vi "Test Different ImageResIDs.vi"(8 "error in (no error)":errorcluster) -> (0 "error out":errorcluster)   [LabVIEW 2026, in "VILab.lvlib"]
uses:
  VILab.lvlib
  SubVIs/Find Resource by Type (String).vi
  CTLs/Resource.ctl
  <vilib>/Utility/traverseref.llb/VI Scripting - Traverse.lvlib
  <vilib>/Utility/traverseref.llb/TRef TravTarget.ctl
panel:
  out "Last Error":errorcluster
  out "Working IDs":i32[](array[numeric])=[0, 1, 2, 3, 4, 5, 6, 7, 8, 9, 10, 11, 12, 13, 14, 15, 16, 17, 18, 19, 20, 21, 22, 23, 24, 25, 26, 27, 28, 29, 30, 31, 32, 33, 34, 35, 36, 37, 38, 39, 40, 41, 42, 43, 44, 45, 46, 47, 48, 49, 50, 51, 52, 53, 54, 55, 56, 57, 58, 59, 60, 61, 62, 63, 64, 65, 66, 67, 68, 69, 70, 71, 72, 73, 74, 75, 76, 77, 78, 79, 80, 81, 82, 83, 84, 85, 86, 87, 88, 89, 90, 91, 92, 93, 94, 95, 96, 97, 98, 99, 100, 101, 102, 103, 104, 105, 106, 107, 108, 109, 110, 111, 112, 113, 114, 115, 116, 117, 118, 119, 120, 121, 122, 123, 124, 125, 126, 127, 128, 129, 130, 131, 132, 133, 134, 135, 136, 137, 138, 139, 140, 141, 142, 143, 144, 145, 146, 147, 148, 149, 150, 151, 152, 153, 154, 155, 156, 157, 158, 159, 160, 161, 162, 163, 164, 165, 166, 167, 168, 169, 170, 171, 172, 173, 174, 175, 176, 177, 178, 179, 180, 181, 182, 183, 184, 185, 186, 187, 188, 189, 190, 191, 192, 193, 194, 195, 196, 197, 198, 199, 200, 201, 202, 203, 204, 205, 206, 207, 208, 209, 210, 211, 212, 213, 214, 215, 216, 217, 218, 219, 220, 221, 222, 223, 224, 225, 226, 227, 228, 229, 230, 231, 238, 239, 240, 241, 242, 243, 244, 245, 246, 247, 248, 249, 250, 251, 252, 253, 254, 255, 256, 257, 258, 259, 260, 261, 262, 263, 264, 265, 266, 267, 268, 269, 270, 271, 272, 273, 274, 275, 276, 277, 278, 279, 280, 281, 282, 283, 284, 285, 286, 287, 288, 289, 290, 291, 292, 293, 294, 295, 296, 297, 298, 299, 300, 301, 302, 303, 304, 305, 306, 307, 308, 309, 310, 311, 312, 313, 314, 315, 316, 317, 318, 319, 320, 321, 322, 323, 324, 325, 326, 327, 328, 329, 330, 331, 332, 333, 334, 335, 336, 337, 338, 339, 340, 341, 342, 343, 344, 345, 346, 347, 348, 349, 350, 351, 352, 353, 354, 355, 356, 357, 358, 359, 360, 361, 362, 363, 364, 365, 366, 373, 374, 375, 376, 377, 378, 379, 380, 381, 382, 383, 384, 385, 386, 387, 388, 389, 390, 391, 393, 394, 395, 396, 397, 398, 399, 400, 401, 402, 403, 404, 405, 406, 407, 408, 409, 410, 411, 412, 413, 414, 415, 416, 417, 418, 419, 420, 421, 422, 423, 424, 425, 426, 427, 428, 429, 430, 431, 432, 433, 434, 435, 436, 437, 438, 439, 440, 441, 442, 443, 444, 445, 446, 447, 448, 449, 450, 451, 452, 453, 454, 455, 456, 457, 458, 459, 460, 461, 462, 463, 464, 465, 466, 467, 468, 469, 470, 471, 472, 473, 474, 475, 476, 477, 478, 479, 480, 481, 482, 483, 484, 485, 486, 487, 488, 489, 490, 491, 492, 493, 494, 495, 496, 497, 498, 499, 500, 505, 506, 507, 508, 509, 510, 511, 512, 513, 514, 515, 516, 517, 518, 519, 520, 521, 522, 523, 524, 525, 526, 527, 528, 529, 530, 531, 533, 534, 535, 536, 537, 538, 539, 540, 541, 543, 544, 545, 546, 547, 548, 549, 550, 551, 552, 553, 554, 555, 556, 557, 558, 559, 560, 561, 562, 563, 564, 565, 566, 567, 568, 569, 570, 571, 572, 573, 574, 575, 576, 577, 578, 579, 580, 581, 582, 583, 584, 585, 586, 587, 588, 589, 590, 591, 592, 593, 594, 595, 596, 597, 598, 599, 600, 601, 602, 603, 604, 605, 606, 607, 608, 609, 610, 611, 612, 613, 614, 615, 616, 617, 618, 619, 620, 621, 622, 623, 624, 625, 626, 627, 628, 629, 630, 631, 632, 633, 634, 635, 636, 637, 638, 639, 640, 641, 644, 645, 648, 649, 650, 651, 652, 653, 654, 655, 656, 657, 658, 659, 660, 661, 662, 663, 664, 665, 666, 667, 668, 669, 670, 671, 672, 673, 674, 675, 676, 677, 678, 679, 680, 681, 682, 683, 684, 685, 686, 687, 688, 689, 690, 691, 692, 693, 694, 695, 696, 697, 698, 699, 700, 701, 702, 703, 704, 705, 706, 707, 708, 709, 710, 711, 712, 713, 714, 715, 716, 717, 718, 719, 720, 721, 722, 723, 724, 725, 726, 727, 728, 729, 730, 731, 732, 733, 734, 735, 736, 737, 738, 739, 740, 741, 742, 743, 744, 745, 746, 747, 748, 749, 750, 751, 752, 753, 754, 755, 756, 757, 758, 759, 760, 761, 762, 763, 764, 766, 767, 768, 769, 771, 772, 773, 774, 775, 776, 777, 778, 779, 780, 781, 782, 783, 786, 787, 788, 789, 790, 791, 792, 793, 794, 795, 796, 797, 798, 799, 800, 801, 802, 803, 804, 805, 806, 807, 808, 809, 810, 811, 812, 813, 814, 815, 816, 817, 818, 819, 820, 821, 822, 823, 824, 825, 826, 827, 828, 829, 830, 831, 832, 833, 834, 835, 836, 837, 838, 839, 1000, 1001, 1002, 1003, 1004, 1005, 1006, 1007, 1008, 1009, 1010, 1011, 1012, 1013, 1014, 1015, 1016, 1017, 1018, 1019, 1020, 1021, 1022, 1023, 1024, 1025, 1026, 1027, 1028, 1029, 1030, 2000, 2001, 2002, 2003, 2004, 2005, 2006, 2007, 2008, 2009, 2010, 2011, 2012, 2013, 2014, 2015, 2016, 2017, 2018, 2019, 2020, 2021, 2022, 2023, 2024, 2025, 2026, 2027, 2028, 2029, 2030, 2031, 2032, 2033, 2034, 2035, 2036, 2037, 2038, 2039, 2040, 2041, 2042, 2043, 2044, 2045, 2046, 2047, 2048, 2049, 2050, 2051, 2052, 2053, 2054, 2055, 2056, 2057, 2058, 2059, 2060, 2061, 2062, 2063, 2064, 2065, 2066, 2067, 2068, 2069, 2070, 2071, 2072, 2073, 2074, 2075, 2076, 2077, 2078, 2079, 2080, 2081, 2082, 2083, 2084, 2085, 2086, 2087, 2088, 2089, 2090, 2091, 2092, 2093, 2094, 2095, 2096, 2097, 2098, 2099, 2100, 2101, 2102, 2103, 2104, 2105, 2106, 2107, 2108, 2109, 3000, 3001, 3002, 3003, 3004, 3005, 3006, 3007, 3008, 3009, 3010, 3011, 3012, 3013, 3014, 3015, 3016, 3017, 3018, 3019, 3020, 3021, 3022, 3023, 3024, 3025, 3026, 3027, 3028, 3029, 3030, 3031, 3032, 3033, 3034, 3035, 3036, 3037, 3038, 3039, 3040, 3041, 3042, 3043, 3044, 3045, 3046, 3047, 3048, 3049, 3050, 3051, 3052, 3053, 3054, 3055, 3056, 3057, 3058, 3059, 3060, 3061, 3062, 3063, 3064, 3065, 3066, 3067, 3068, 3069, 3070, 3071, 3072, 3073, 3074, 3075, 3076, 3077, 3078, 3079, 3080, 3081, 3082, 3083, 3084, 3085, 3086, 3087, 3088, 3089, 3090, 3091]
  out "i":i32
  in  "stop":bool
  # "tried up to -5000"
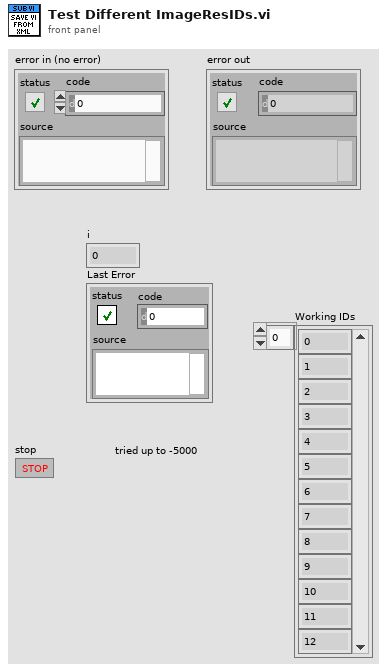
[diagram p1: front panel]
types:
  T1 = typedef "TRef TravTarget.ctl" = enum16{"FP", "BD", "Other"}
  T2 = typedef "VILab.lvlib/Resource.ctl" = cluster{"type":u32, "id":i32, "name":string, "binary data":string}
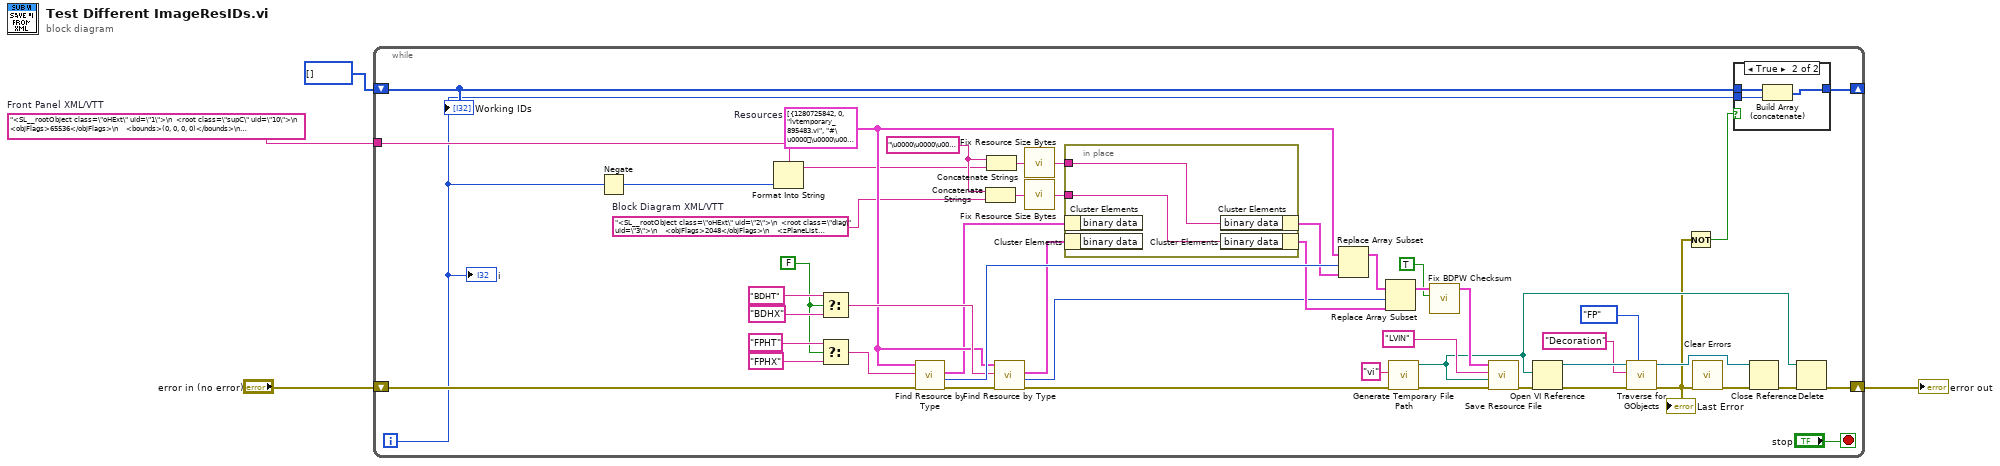
[diagram p0: block diagram]
diagram:
  w2 = "<SL__rootObject class=\"oHExt\" uid=\"1\">\n  <root class=\"supC\" uid=\"10\">\n    <objFlags>65536</objFlags>\n    <bounds>(0, 0, 0, 0)</bounds>\n    <MouseWheelSupport>0</MouseWheelSupport>\n    <ddoList elements=\"0\">\n      </ddoList>\n    <paneHierarchy class=\"pane\" uid=\"12\">\n      <objFlags>2492464</objFlags>\n      <howGrow>240</howGrow>\n      <bounds>(46, 0, 668, 1090)</bounds>\n      <partsList elements=\"6\">\n        <SL__arrayElement class=\"label\" uid=\"15\">\n          <objFlags>1511754</objFlags>\n          <partID>16</partID>\n          <masterPart>28</masterPart>\n          <howGrow>5</howGrow>\n          <bounds>(0, 0, 17, 29)</bounds>\n          <image class=\"Image\">\n            <ImageResID>-9</ImageResID>\n            </image>\n          <fgColor>01000000</fgColor>\n          <bgColor>01000000</bgColor>\n          <textRec class=\"textHair\">\n            <mode>1028</mode>\n            <text>\"Pane\"</text>\n            <bgColor>01000000</bgColor>\n            </textRec>\n          </SL__arrayElement>\n        <SL__arrayElement class=\"cosm\" uid=\"16\">\n          <objFlags>3442</objFlags>\n          <partID>39</partID>\n          <masterPart>28</masterPart>\n          <howGrow>194</howGrow>\n          <bounds>(0, 1073, 605, 1090)</bounds>\n          <image class=\"Image\">\n            <ImageResID>0</ImageResID>\n            </image>\n          <bgColor>00B3B3B3</bgColor>\n          </SL__arrayElement>\n        <SL__arrayElement class=\"cosm\" uid=\"17\">\n          <objFlags>3442</objFlags>\n          <partID>38</partID>\n          <masterPart>28</masterPart>\n          <howGrow>56</howGrow>\n          <bounds>(605, 0, 622, 1073)</bounds>\n          <image class=\"Image\">\n            <ImageResID>0</ImageResID>\n            </image>\n          <bgColor>00B3B3B3</bgColor>\n          </SL__arrayElement>\n        <SL__arrayElement class=\"cosm\" uid=\"18\">\n          <objFlags>7539</objFlags>\n          <partID>44</partID>\n          <masterPart>28</masterPart>\n          <howGrow>10</howGrow>\n          <bounds>(605, 1073, 622, 1090)</bounds>\n          <image class=\"Image\">\n            <ImageResID>-365</ImageResID>\n            </image>\n          <fgColor>00B3B3B3</fgColor>\n          <bgColor>00B3B3B3</bgColor>\n          </SL__arrayElement>\n        <SL__arrayElement class=\"cosm\" uid=\"19\">\n          <objFlags>4211</objFlags>\n          <partID>28</partID>\n          <howGrow>120</howGrow>\n          <bounds>(0, 0, 605, 1073)</bounds>\n          <image class=\"Image\">\n            <ImageResID>-704</ImageResID>\n            </image>\n          <fgColor>00E2E2E2</fgColor>\n          <bgColor>00E2E2E2</bgColor>\n          </SL__arrayElement>\n        <SL__arrayElement class=\"annex\" uid=\"20\">\n          <partID>66</partID>\n          </SL__arrayElement>\n        </partsList>\n      <paneFlags>331089</paneFlags>\n      <minPaneSize>(1,1)</minPaneSize>\n      <docBounds>(-127, -244, 605, 1073)</docBounds>\n      <zPlaneList elements=\"1\">\n        <SL__arrayElement class=\"cosm\" uid=\"52\">\n          <objFlags>3</objFlags>\n          <bounds>(-22, 24, 10, 56)</bounds>\n          <image class=\"Image\">\n            <ImageResID>%d</ImageResID>\n            </image>\n          <fgColor>00A8ABAE</fgColor>\n          <bgColor>00FFFFFF</bgColor>\n          </SL__arrayElement>\n        </zPlaneList>\n      <image class=\"Image\">\n        <ImageResID>0</ImageResID>\n        </image>\n      </paneHierarchy>\n    <savedSize>(0, 0, 0, 0)</savedSize>\n    <conPane class=\"conPane\" uid=\"21\">\n      <conId>4815</conId>\n      <cons elements=\"12\">\n        </cons>\n      </conPane>\n    <keyMappingList class=\"keyMapList\" uid=\"22\">\n      </keyMappingList>\n    </root>\n  <pBounds>(46, 0, 668, 1090)</pBounds>\n  <dBounds>(0, 0, 0, 0)</dBounds>\n  <origin>(723,351)</origin>\n  <instrStyle>31</instrStyle>\n  <blinkList elements=\"0\">\n    </blinkList>\n  </SL__rootObject>\n"  # Front Panel XML/VTT
  n1 = while {
    shift-right: [w13] -> w3
    shift-left: "error in (no error)" -> [w30]
    tunnel: w2 -> [w24]
    shift-right: [w20] -> _
    shift-left: i32[] [] -> [w22]
    i -> [w21]
    stop <- "stop" stop-if-true
    w28 = FALSE ("Use VTT?")
    w26 = "<SL__rootObject class=\"oHExt\" uid=\"2\">\n  <root class=\"diag\" uid=\"3\">\n    <objFlags>2048</objFlags>\n    <zPlaneList elements=\"0\">\n      </zPlaneList>\n    <nodeList elements=\"1\">\n      <SL__arrayElement class=\"sRN\" uid=\"7\">\n        <termList elements=\"0\">\n          </termList>\n        <bounds>(0, 0, 0, 0)</bounds>\n        <shortCount>1</shortCount>\n        <clumpNum>131075</clumpNum>\n        </SL__arrayElement>\n      </nodeList>\n    <signalList elements=\"0\">\n      </signalList>\n    <bgColor>00FFFFFF</bgColor>\n    <firstNodeIdx>1</firstNodeIdx>\n    </root>\n  <pBounds>(46, 0, 651, 1073)</pBounds>\n  <dBounds>(46, 0, 651, 1073)</dBounds>\n  <origin>(1124,436)</origin>\n  <instrStyle>31</instrStyle>\n  </SL__rootObject>\n"  # Block Diagram XML/VTT
    w27 = T2[] [{"type"=1280725842, "id"=0, "name"="lvtemporary_895483.vi", "binary data"="#\u0000\u0000\u0000\u0000\u0000\u0000 \u0000\u0006\u0000\u0000\u0000\u0000\u0004\u0000\u0003\u0000<\u0000\u0000\u0000\u001f@\u0002\u0000\u0000\u0000\u0000\u0001\u0000\u0001\u0000\u0002ÿÿÿÿ\u0000\u0000\u0000\u0000\u0000\u0000\u0000\u0000\u0000\u0000\u0000\u0000\u0000\u0000\u0000\u0000\u0000\u0000\u0000\u0000\u0000\u0000\u0000\u0000\u0000\u0000\u0000\u0000\u0000\u0000\u0000\f\u0000\u0000\u0000\u0010\u0000\u0000\u0000\u0000\u0000\u0000\u0000\u0000\u0000\u0000\u0000\u0000\u0000\u0000\u0000\u0000\u0000\u0000\u0000\u0000Ô\u001dÙ\u0000²\u0004é\tìøB~\u0000\u0000\u0000\u0000\u0000\u0000\u0000\u0000\u0000\u0000\u0000\u0000\u0000\u0000\u0000\u0000\u0000\u0000\u0000\u0000\u0000\u0000\u0000\u0000\u0001\u0000\u0000\u0000ÿÿÿÿÔ\u001dÙ\u0000²\u0004é\tìøB~"}, {"type"=1381258055, "id"=0, "name"="", "binary data"="\u0000\u0000\u0000\u0000\u0000\u0000\u0000\u0000\u0000\u0000\u0000\u0000\u0000\u0000\u0000\u0000"}, {"type"=1986359923, "id"=4, "name"="", "binary data"="#6€\u0006\u0000\u0000\u000623.3.6\u0000"}, {"type"=1129270864, "id"=0, "name"="", "binary data"="\u0000\u0001"}, {"type"=1279882857, "id"=0, "name"="", "binary data"="\u0000\u0001LVIN\u0000\u0000\u0000\u0000\u0000\u0003"}, {"type"=1111773271, "id"=0, "name"="", "binary data"="Ô\u001dÙ\u0000²\u0004é\tìøB~K@I.b\u0001-\u001amå­U\u0006òv\u001f\n¦©fí²\u0002\u0013@î¼ "}, {"type"=1229147982, "id"=0, "name"="", "binary data"="ÿÿÿÿ\u0000\u0000\u0001\u0000\u0000\u0001ÿü\u0001\u0000T\u0001ÿT\u0001ûT\u0001u\u0004\u0001u$\u0001®T\u0001®T\u0001ß$\u0001ÿ\u0004\u0001\u0000\u001c\u0001\u0000\u0016\u0001\u0010ñ;\u0012a$\u0017\u001dÿòaIñ2\u0016\u0001\u0018\u0001x\u0000\u0001\u0000\u0000\u0001\u0000\u0000\u0001\u0000\u0000\u0001\u0000\u0000\u0001\u0000\u0000\u0001\u0000\u0000\u0001\u0000\u0000\u0001\u0000\u0000\u0001ÿÿÿÿ"}, {"type"=1768123448, "id"=0, "name"="", "binary data"="ÿÿÿÿÿÿÿÿÿÿÿÿÿÿÿÿÿÿÿÿÿÿÿÿÿÿÿÿÿÿÿÿÿ\u0000\u0000\u0000\u0000\u0000\u0000\u0000\u0000\u0000\u0000\u0000\u0000\u0000\u0000\u0000\u0000\u0000\u0000\u0000\u0000\u0000\u0000\u0000\u0000\u0000\u0000\u0000\u0000\u0000\u0000ÿÿ\u0000\u0000\u0000\u0000\u0000\u0000\u0000\u0000\u0000\u0000\u0000\u0000\u0000\u0000\u0000\u0000\u0000\u0000\u0000\u0000\u0000\u0000\u0000\u0000\u0000\u0000\u0000\u0000\u0000\u0000ÿÿ\u0000\u0000ÿÿÿÿÿÿÿÿÿÿÿÿÿÿÿÿÿÿÿ\u0000\u0000\u0000\u0000\u0000\u0000\u0000\u0000\u0000ÿÿ\u0000\u0000ÿùùùùùùùùùùùù÷ù,ù,à\u0000\u0000\u0000\u0000\u0000\u0000\u0000\u0000\u0000ÿÿ\u0000\u0000ÿùÿÿÿÿÿÿÿÿÿÿÿ÷ù,ù,ÿ\u0000\u0000\u0000\u0000\u0000\u0000\u0000\u0000\u0000ÿÿ\u0000\u0000ÿùÿèäèÿÿÿèäèÿ÷ü+ü,ÿ\u0000\u0000\u0000\u0000\u0000\u0000\u0000\u0000\u0000ÿÿ\u0000\u0000ÿùÿäÿäÿÿÿäÿäÿ÷,,,,à\u0000\u0000\u0000\u0000\u0000\u0000\u0000\u0000\u0000ÿÿ\u0000\u0000ÿùèäÿäèÿèäÿäè÷+ü+,ÿ\u0000\u0000\u0000\u0000\u0000\u0000\u0000\u0000\u0000ÿÿ\u0000\u0000ÿùäèÿèäÿäèÿèä÷ü\bü,ÿ\u0000\u0000\u0000\u0000\u0000\u0000\u0000\u0000\u0000ÿÿ\u0000\u0000ÿùäÿÿÿäÿäÿÿÿä÷ü\bü,ÿ\u0000\u0000\u0000\u0000\u0000\u0000\u0000\u0000\u0000ÿÿ\u0000\u0000ÿùÿÿÿÿèäèÿÿÿÿ÷+ü+,ÿ\u0000\u0000\u0000\u0000\u0000\u0000\u0000\u0000\u0000ÿÿ\u0000\u0000ÿùÿÿÿÿÿÿÿÿÿÿÿ÷,,,,ÿ\u0000\u0000\u0000\u0000\u0000\u0000\u0000\u0000\u0000ÿÿ\u0000\u0000ÿ÷÷÷÷÷÷÷÷÷÷÷÷÷,,ƒƒÿ\u0000\u0000\u0000\u0000\u0000\u0000\u0000\u0000\u0000ÿÿ\u0000\u0000ÿ,,,,,,,,,,,,,,,ƒ\u0005ƒƒ\u0000\u0000\u0000\u0000\u0000\u0000\u0000\u0000ÿÿ\u0000\u0000ÿ,ü,,,,,ü,,,,###ƒ\u0005\u0005\u0005ƒƒ\u0000\u0000\u0000\u0000\u0000\u0000ÿÿ\u0000\u0000ÿüðü,,,ü#ü,##,,,ƒ\u0005\u0005ÿ\u0005\u0005ƒƒ\u0000\u0000\u0000\u0000ÿÿ\u0000\u0000ÿ,ï,,,,#,,#,,,,,ƒ\u0005ÿÿÿ\u0005\u0005\u0005ƒ##\u0000ÿÿ\u0000\u0000ÿÿðÿÿÿ#ÿÿ#ÿÿÿÿÿÿƒ\u0005\u0005ÿ\u0005..."}, {"type"=1414091852, "id"=0, "name"="", "binary data"="\tSource VI"}, {"type"=1129333554, "id"=0, "name"="", "binary data"="\u0000\u0001"}, {"type"=1279878768, "id"=0, "name"="", "binary data"="\u0000\u0001FPHP\u0000\u0000\u0000\u0000\u0000\u0003"}, {"type"=1179665784, "id"=0, "name"="", "binary data"="\u0000\u0000\u0000\u0000"}, {"type"=1179666520, "id"=0, "name"="", "binary data"="\u0000\u0000\u000eØ<SL__rootObject class=\"oHExt\" uid=\"1\">\n  <root class=\"supC\" uid=\"10\">\n    <objFlags>65536</objFlags>\n    <bounds>(0, 0, 0, 0)</bounds>\n    <MouseWheelSupport>0</MouseWheelSupport>\n    <ddoList elements=\"0\">\n      </ddoList>\n    <paneHierarchy class=\"pane\" uid=\"12\">\n      <objFlags>2492464</objFlags>\n      <howGrow>240</howGrow>\n      <bounds>(46, 0, 668, 1090)</bounds>\n      <partsList elements=\"6\">\n        <SL__arrayElement class=\"label\" uid=\"15\">\n          <objFlags>1511754</objFlags>\n          <partID>16</partID>\n          <masterPart>28</masterPart>\n          <howGrow>5</howGrow>\n          <bounds>(0, 0, 17, 29)</bounds>\n          <image class=\"Image\">\n            <ImageResID>-9</ImageResID>\n            </image>\n          <fgColor>01000000</fgColor>\n          <bgColor>01000000</bgColor>\n          <textRec class=\"textHair\">\n            <mode>1028</mode>\n            <text>\"Pane\"</text>\n            <bgColor>01000000</bgColor>\n            </textRec>\n          </SL__arrayElement>\n        <SL__arrayElement class=\"cosm\" uid=\"16\">\n          <objFlags>3442</objFlags>\n          <partID>39</partID>\n          <masterPart>28</masterPart>\n          <howGrow>194</howGrow>\n          <bounds>(0, 1073, 605, 1090)</bounds>\n          <image class=\"Image\">\n            <ImageResID>0</ImageResID>\n            </image>\n          <bgColor>00B3B3B3</bgColor>\n          </SL__arrayElement>\n        <SL__arrayElement class=\"cosm\" uid=\"17\">\n          <objFlags>3442</objFlags>\n          <partID>38</partID>\n          <masterPart>28</masterPart>\n          <howGrow>56</howGrow>\n          <bounds>(605, 0, 622, 1073)</bounds>\n          <image class=\"Image\">\n            <ImageResID>0</ImageResID>\n            </image>\n          <bgColor>00B3B3B3</bgColor>\n          </SL__arrayElement>\n        <SL__arrayElement class=\"cosm\" uid=\"18\">\n          <objFlags>7539</objFlags>\n          <partID>44</partID>\n          <masterPart>28</masterPart>\n          <howGrow>10</howGrow>\n          <bounds>(605, 1073, 622, 1090)</bounds>\n          <image class=\"Image\">\n            <ImageResID>-365</ImageResID>\n            </image>\n          <fgColor>00B3B3B3</fgColor>\n          <bgColor>00B3B3B3</bgColor>\n          </SL__arrayElement>\n        <SL__arrayElement class=\"cosm\" uid=\"19\">\n          <objFlags>4211</objFlags>\n          <partID>28</partID>\n          <howGrow>120</howGrow>\n          <bounds>(0, 0, 605, 1073)</bounds>\n          <image class=\"Image\">\n            <ImageResID>-704</ImageResID>\n            </image>\n          <fgColor>00E2E2E2</fgColor>\n          <bgColor>00E2E2E2</bgColor>\n          </SL__arrayElement>\n        <SL__arrayElement class=\"annex\" uid=\"20\">\n          <partID>66</partID>\n          </SL__arrayElement>\n        </partsList>\n      <paneFlags>331089</paneFlags>\n      <minPaneSize>(1,1)</minPaneSize>\n      <docBounds>(-127, -244, 605, 1073)</docBounds>\n      <zPlaneList elements=\"1\">\n        <SL__arrayElement class=\"cosm\" uid=\"52\">\n          <objFlags>3</objFlags>\n          <bounds>(-22, 24, 10, 56)</bounds>\n          <image class=\"Image\">\n            <ImageResID>-11</ImageResID>\n            </image>\n          <fgColor>00A8ABAE</fgColor>\n          <bgColor>00FFFFFF</bgColor>\n          </SL__arrayElement>\n        </zPlaneList>\n      <image class=\"Image\">\n        <ImageResID>0</ImageResID>\n        </image>\n      </paneHierarchy>\n    <savedSize>(0, 0, 0, 0)</savedSize>\n    <conPane class=\"conPane\" uid=\"21\">\n      <conId>4815</conId>\n      <cons elements=\"12\">\n        </cons>\n      </conPane>\n    <keyMappingList class=\"keyMapList\" uid=\"22\">\n      </keyMappingList>\n    </root>\n  <pBounds>(46, 0, 668, 1090)</pBounds>\n  <dBounds>(0, 0, 0, 0)</dBounds>\n  <origin>(723,351)</origin>\n  <instrStyle>31</instrStyle>\n  <blinkList elements=\"0\">\n    </blinkList>\n  </SL__rootObject>\n"}, {"type"=1179669317, "id"=0, "name"="", "binary data"="\u0000\u0000\u0000\u0010"}, {"type"=1448100944, "id"=0, "name"="", "binary data"="\u0000\u0000\u0000\u0000"}, {"type"=1279877732, "id"=0, "name"="", "binary data"="\u0000\u0001BDHP\u0000\u0000\u0000\u0000\u0000\u0003"}, {"type"=1111770488, "id"=0, "name"="", "binary data"="\u0000\u0000\u0000\u0000"}, {"type"=1111771224, "id"=0, "name"="", "binary data"="\u0000\u0000\u0002Ð<SL__rootObject class=\"oHExt\" uid=\"2\">\n  <root class=\"diag\" uid=\"3\">\n    <objFlags>2048</objFlags>\n    <zPlaneList elements=\"0\">\n      </zPlaneList>\n    <nodeList elements=\"1\">\n      <SL__arrayElement class=\"sRN\" uid=\"7\">\n        <termList elements=\"0\">\n          </termList>\n        <bounds>(0, 0, 0, 0)</bounds>\n        <shortCount>1</shortCount>\n        <clumpNum>131075</clumpNum>\n        </SL__arrayElement>\n      </nodeList>\n    <signalList elements=\"0\">\n      </signalList>\n    <bgColor>00FFFFFF</bgColor>\n    <firstNodeIdx>1</firstNodeIdx>\n    </root>\n  <pBounds>(46, 0, 651, 1073)</pBounds>\n  <dBounds>(46, 0, 651, 1073)</dBounds>\n  <origin>(1124,436)</origin>\n  <instrStyle>31</instrStyle>\n  </SL__rootObject>\n"}, {"type"=1111774021, "id"=0, "name"="", "binary data"="\u0000\u0000\u0000\u0007"}, {"type"=1447646291, "id"=0, "name"="", "binary data"="\u0000\u0000\u0000\u0001\u0000\u0000\u0000\u0014NI.LV.All.SourceOnly\u0000\u0000\u0000\u0015#\u0000€\u0000\u0000\u0000\u0000\u0001\u0000\u0004\u0000!\u0000\u0001\u0000\u0000\u0001\u0000\u0000\u0000\u0000"}, {"type"=1146374224, "id"=0, "name"="", "binary data"="\u0000\u0000"}, {"type"=1297434948, "id"=0, "name"="", "binary data"="\u0000\u0000\u00004"}, {"type"=1212765012, "id"=0, "name"="", "binary data"="\u0000\u0000\u0000\u0002\u0000\u0000\u0004\u0000\u0000\u0000\u0000\u0002\u0000\u0000\u0000\u0000\u0000\u0000\u0000\u0000\u0000\u0000\u0000\u0000\u0000\u0000\u0000\u0000\u0000\u0000\u0000\u0000\u0000\u0000\u0000\u0000\u0000\u0000\u0000\u0000"}, {"type"=1447253072, "id"=0, "name"="", "binary data"="\u0000\u0000\u0000`xœc```b`a``\baøÀÀÃ€\u001bTà‘Ã\u0005\u0018\u0019\u0018\u0001Œr\u0001Ñ"}, {"type"=1179926850, "id"=128, "name"="", "binary data"="\u0000\u0001\u0000\u0002\u0000\u0003\u0000\u0004\u0000\u0000\u0000H\u0000\u000f\u0004\u0000\u0000\u0000\u0000\u000f\u0000Ù\u0000Ô\u0000\u0000\u0000Q\u0000\u000f\u0004\u0000\u0000\u0000\u0000\u000f\u0000Ù\u0000Ô\u0000\u0000\u0000Z\u0000\u000f\u0004\u0000\u0000\u0000\u0000\u000f\u0000Ù\u0000Ô\u0000\u0000\u0000c€\u0000„\u0000€\u0000\u0000\u000f\u0000Ù\u0000Ô\bSegoe UI\bSegoe UI\bSegoe UI\u00010"}]  # Resources
    w53 = "\u0000\u0000\u0000\u0000"
    n2 = Negate(x=w21) -> (-x=w7:i32)
    n3 = Format Into String(format string=w24, w7) -> (resulting string=w23:string)  [unwired: 2 in, 1 out]
    n4 = Select(t="BDHT", s=w28, f="BDHX") -> (s? t:f=w29:string)
    n5 = Select(t="FPHT", s=w28, f="FPHX") -> (s? t:f=w34:string)
    n6 = call-poly "Find Resource by Type.vi"("error in (no error)"=w30, "Resource Type"=w34, "Resources"=w27) -> ("error out"=w31:errorcluster, "Index"=w48:i32, "Resource"=w6:T2)  [unwired: 4 in, 2 out]
    n7 = Concatenate Strings(w53, w26) -> (w51:string)
    n8 = Concatenate Strings(w53, w23) -> (w52:string)
    n9 = call-poly "Find Resource by Type.vi"("error in (no error)"=w31, "Resource Type"=w29, "Resources"=w27) -> ("error out"=w32:errorcluster, "Index"=w45:i32, "Resource"=w5:T2)  [unwired: 4 in, 2 out]
    n10 = call "Fix Resource Size Bytes.vi"("Data in"=w52) -> ("Data out"=w50:string)
    n11 = call "Fix Resource Size Bytes.vi"("Data in"=w51) -> ("Data out"=w49:string)
    n12 = in-place {
      in-place-border: w50 -> [w59]
      in-place-border: w49 -> [w58]
      n13 = in-place-cluster #1(w6) -> ()  [unwired: 1 out]
      n14 = in-place-cluster #2(w5) -> ()  [unwired: 1 out]
      n15 = in-place-cluster #1("binary data"=w59) -> (w47:T2)
      n16 = in-place-cluster #2("binary data"=w58) -> (w46:T2)
    }
    n17 = Replace Array Subset(array=w27, new element=w47, index=w48) -> (w44:T2[])
    n18 = Replace Array Subset(array=w44, new element=w46, index=w45) -> (w42:T2[])
    n19 = call <vilib>:"Generate Temporary File Path.vi"("error in (no error)"=w32, "Temporary File Extension (tmp)"="vi") -> ("error out"=w33:errorcluster, "Unique Temporary File Path"=w9:path)  [unwired: 8 in]
    n20 = call "Fix BDPW Checksum.vi"("Only fix 3rd hash (F)"=TRUE, "Resources"=w42) -> ("Resources out"=w41:T2[])  [unwired: 8 in, 1 out]
    n21 = call "Save Resource File.vi"("error in (no error)"=w33, "Path"=w9, "File type"="LVIN", "Resources"=w41) -> ("error out"=w14:errorcluster)  [unwired: 7 in]
    n22 = Open VI Reference(vi path=w9, error in (no error)=w14) -> (vi reference=w18:refnum<vi>, error out=w17:errorcluster)  [unwired: 4 in]
    n23 = call <vilib>:"Traverse for GObjects.vi"("Traverse Target"=TRef_TravTarget."FP", "error in (no error)"=w17, "Class Name"="Decoration", "VI Refnum"=w18) -> ("error out"=w8:errorcluster, "dup VI Refnum"=w10:refnum<vi>)  [unwired: 4 in, 2 out]
    "Last Error" <- w8
    n24 = Not(x=w8) -> (.not. x?=w19:bool)
    n25 = call <vilib>:"Clear Errors.vi"("error in (no error)"=w8) -> ("error out"=w11:errorcluster)  [unwired: 5 in, 1 out]
    n26 = case shown="True" w19 {
      tunnel: w22 -> [w54 w57]
      tunnel: w21 -> [_ w56]
      tunnel: [w54 w55] -> w20
      frame False {
      }
      frame True {
        n27 = Build Array (concatenate)(w57, w56) -> (w55:i32[])
      }
    }
    n28 = Close Reference(reference=w10, error in (no error)=w11) -> (error out=w12:errorcluster)
    n29 = Delete(path (use dialog)=w9, error in=w12) -> (error out=w13:errorcluster)  [unwired: 3 in, 2 out]
    "i" <- w21
    "Working IDs" <- w22
  }
  "error out" <- w3
